vi "Configure Async Message.vi"(9 "SubAddress":T1=enum."1", 10 "Terminal Address":T2, 11 "Async Command Type":T3) -> (3 "Async Message":refnum<class "Async Message.lvclass">)   [LabVIEW 2020, in "BCI-1553 RealTime API Examples.lvlib"]
uses:
  BCI-1553 RealTime API Examples.lvlib
  src/RealTime/Frames & Messages/Async Message/Async Message.lvclass
  src/RealTime/Frames & Messages/TypeDefs/Command Type.ctl
  src/RealTime/Frames & Messages/TypeDefs/Command Terminal Address.ctl
  src/RealTime/Frames & Messages/TypeDefs/Command SubAddress.ctl
  src/RealTime/Frames & Messages/TypeDefs/Async Message Config.ctl
  src/RealTime/Frames & Messages/TypeDefs/Command Config.ctl
  src/RealTime/Frames & Messages/TypeDefs/Command Word Count.ctl
  src/RealTime/Frames & Messages/TypeDefs/Message Control.ctl
  src/RealTime/Frames & Messages/TypeDefs/Simplified Parameter Data Table.ctl
  src/RealTime/Frames & Messages/TypeDefs/Scaling Information.ctl
  src/RealTime/BCI-1553 API.lvlib
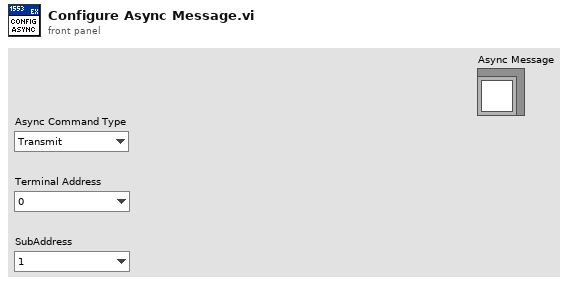
[diagram p1: front panel]
types:
  T1 = typedef "BCI-1553 API.lvlib/Command SubAddress.ctl" = enum16{"Mode Code", "1", "2", "3", "4", "5", "6", "7", "8", "9", "10", "11", "12", "13", "14", "15", "16", "17", "18", "19", "20", "21", "22", "23", "24", "25", "26", "27", "28", "29", "30"}
  T2 = typedef "BCI-1553 API.lvlib/Command Terminal Address.ctl" = enum16{"0", "1", "2", "3", "4", "5", "6", "7", "8", "9", "10", "11", "12", "13", "14", "15", "16", "17", "18", "19", "20", "21", "22", "23", "24", "25", "26", "27", "28", "29", "30", "Broadcast"}
  T3 = typedef "BCI-1553 API.lvlib/Command Type.ctl" = enum16{"Transmit", "Receive"}
  T4 = typedef "BCI-1553 API.lvlib/Simplified Parameter Data Table.ctl" = cluster{"Parameter Name":string, "Base Word":u16, "Scaling Info":T5}
  T5 = typedef "BCI-1553 API.lvlib/Scaling Information.ctl" = cluster{"Bit Offset":i32, "Bit Count":i32, "LSB Resolution":dbl, "2's Complement":bool, "Big Endian":bool, "Sign Bit":bool}
  T6 = typedef "BCI-1553 API.lvlib/Command Word Count.ctl" = enum16{"1", "2", "3", "4", "5", "6", "7", "8", "9", "10", "11", "12", "13", "14", "15", "16", "17", "18", "19", "20", "21", "22", "23", "24", "25", "26", "27", "28", "29", "30", "31", "32"}
  T7 = typedef "BCI-1553 API.lvlib/Message Control.ctl" = cluster{"MC17 Time Sync":bool, "Error Mask":bool, "Service Request Mask":bool, "Busy Mask":bool, "SubSystem Flag Mask":bool, "Terminal Flag Mask":bool, "Reserved Mask":bool, "Retry":bool, "Bus A / !Bus B":bool, "Self-Test Loopback":bool, "Broadcast Mask":bool, "EoM Interrupt":bool, "Mode Code Format":bool, "Broadcast Format":bool, "RT-RT Format":bool}
  T8 = typedef "BCI-1553 API.lvlib/Async Message Config.ctl" = cluster{"Group":i32, "High Priority":bool, "Time to Next Msg (100 us)":u16, "Command Config":T9, "Message Control":T7}
  T9 = typedef "BCI-1553 API.lvlib/Command Config.ctl" = cluster{"Command Type":T3, "Terminal Address":T2, "SubAddress":T1, "Word Count\\Mode Code":T6, "Command Data":u16[]}
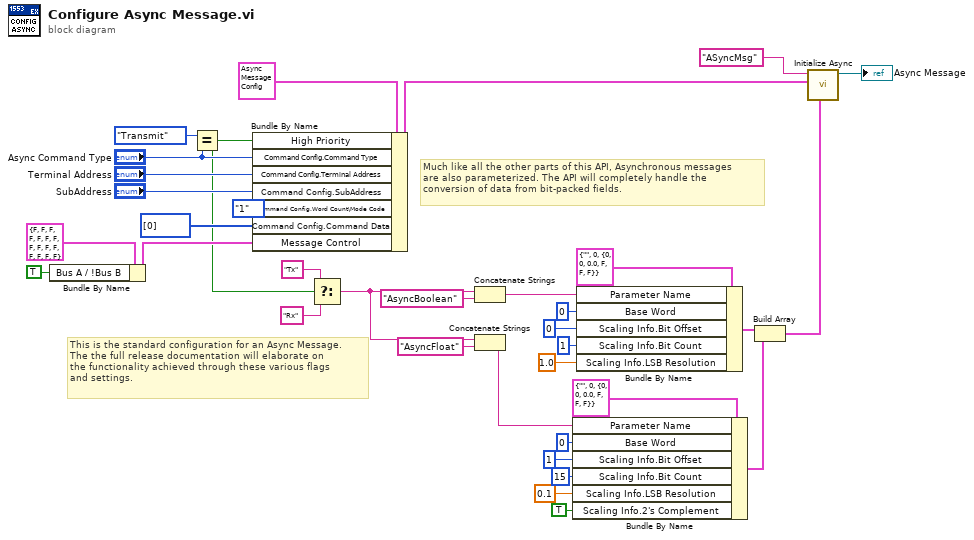
[diagram p0: block diagram]
diagram:
  # "Much like all the other parts of this API, Asynchronous messages\nare also parameterized. The API will completely handle the \nconversion of data from bit-packed fields."
  # "This is the standard configuration for an Async Message.\nThe the full release documentation will elaborate on\nthe functionality achieved through these various flags\nand settings."
  n1 = Bundle By Name(cluster=T7 {"MC17 Time Sync"=FALSE, "Error Mask"=FALSE, "Service Request Mask"=FALSE, "Busy Mask"=FALSE, "SubSystem Flag Mask"=FALSE, "Terminal Flag Mask"=FALSE, "Reserved Mask"=FALSE, "Retry"=FALSE, "Bus A / !Bus B"=FALSE, "Self-Test Loopback"=FALSE, "Broadcast Mask"=FALSE, "EoM Interrupt"=FALSE, "Mode Code Format"=FALSE, "Broadcast Format"=FALSE, "RT-RT Format"=FALSE} ("Message Control"), "Bus A / !Bus B"=TRUE) -> (w30:T7)
  n2 = Equal?(x=Command_Type."Transmit", y="Async Command Type") -> (x = y?=w17:bool)
  n3 = Bundle By Name(cluster=T8 {"Group"=0, "High Priority"=FALSE, "Time to Next Msg (100 us)"=0, "Command Config"={"Command Type"=enum."Transmit", "Terminal Address"=enum."0", "SubAddress"=enum."1", "Word Count\\Mode Code"=enum."1", "Command Data"=[]}, "Message Control"={"MC17 Time Sync"=FALSE, "Error Mask"=FALSE, "Service Request Mask"=FALSE, "Busy Mask"=FALSE, "SubSystem Flag Mask"=FALSE, "Terminal Flag Mask"=FALSE, "Reserved Mask"=FALSE, "Retry"=FALSE, "Bus A / !Bus B"=FALSE, "Self-Test Loopback"=FALSE, "Broadcast Mask"=FALSE, "EoM Interrupt"=FALSE, "Mode Code Format"=FALSE, "Broadcast Format"=FALSE, "RT-RT Format"=FALSE}} ("Async Message Config"), "High Priority"=w17, "Command Config.Command Type"="Async Command Type", "Command Config.Terminal Address"="Terminal Address", "Command Config.SubAddress"="SubAddress", "Command Config.Word Count\\Mode Code"=Command_Word_Count."1" ("Command Config.Word Count"), "Command Config.Command Data"=u16[] [0], "Message Control"=w30) -> (w32:T8)
  n4 = Select(t="Tx" ("Parameter Name"), s=w17, f="Rx" ("Parameter Name")) -> (s? t:f=w20:string)
  n5 = Concatenate Strings(w20, "AsyncBoolean" ("Parameter Name")) -> (w16:string)
  n6 = Concatenate Strings(w20, "AsyncFloat" ("Parameter Name")) -> (w5:string)
  n7 = Bundle By Name(cluster=T4 {"Parameter Name"="", "Base Word"=0, "Scaling Info"={"Bit Offset"=0, "Bit Count"=0, "LSB Resolution"=0.0, "2's Complement"=FALSE, "Big Endian"=FALSE, "Sign Bit"=FALSE}} ("Parameter Table Data"), "Parameter Name"=w5, "Base Word"=u16 0, "Scaling Info.Bit Offset"=1, "Scaling Info.Bit Count"=15, "Scaling Info.LSB Resolution"=0.1, "Scaling Info.2's Complement"=TRUE) -> (w6:T4)
  n8 = Bundle By Name(cluster=T4 {"Parameter Name"="", "Base Word"=0, "Scaling Info"={"Bit Offset"=0, "Bit Count"=0, "LSB Resolution"=0.0, "2's Complement"=FALSE, "Big Endian"=FALSE, "Sign Bit"=FALSE}} ("Parameter Table Data"), "Parameter Name"=w16, "Base Word"=u16 0, "Scaling Info.Bit Offset"=0, "Scaling Info.Bit Count"=1, "Scaling Info.LSB Resolution"=1.0) -> (w7:T4)
  n9 = Build Array(w7, w6) -> (w1:T4[])
  n10 = call "Initialize Async.vi"("Parameters"=w1, "Async Message Config"=w32, "ID"="ASyncMsg") -> ("Async Message out"=→"Async Message":refnum<class "Async Message.lvclass">)  [unwired: 7 in, 1 out]
